vi "DG1022Z DVR.vi"(8 "error in (no error)":errorcluster, 10 "write buffer":string, 11 "VISA resource name":refnum<visa-resource-name>) -> (0 "error out":errorcluster, 2 "read buffer":string)   [LabVIEW 2025, in "Interface Functions.lvlib"]
uses:
  Interface Functions.lvlib
  <vilib>/Instr/_visa.llb/VISA Open Access Mode.ctl
  80e2d14e-0af9-4134-9fdb-927d146bfa2f.vi
  <vilib>/Utility/error.llb/Trim Whitespace One-Sided.vi
panel:
  out "Retries":i32
  out "read return count":u32
  out "write return count":u32
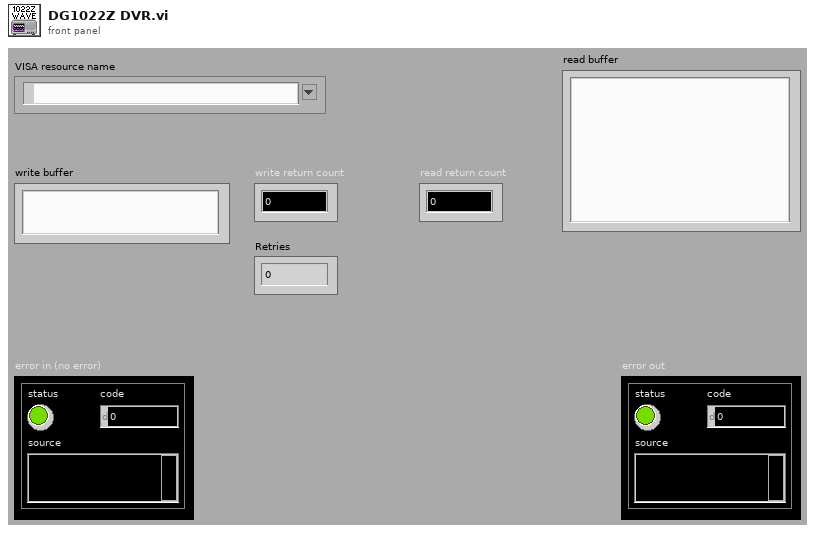
[diagram p1: front panel]
types:
  T1 = typedef "VISA Open Access Mode.ctl" = u32
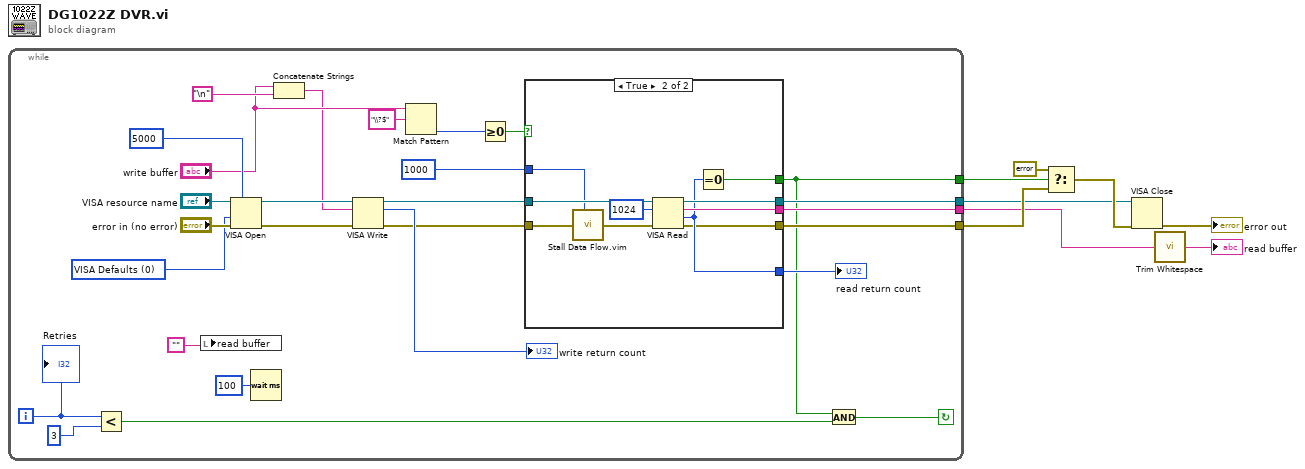
[diagram p0: block diagram]
diagram:
  n1 = while {
    tunnel: [w22] -> w5
    tunnel: [w14] -> w4
    tunnel: [w21] -> w3
    tunnel: [w18] -> w1
    i -> [w16]
    stop <- w12 continue-if-true
    w33 = T1 0 items=["VISA Defaults"=0, "Exclusive Lock"=1, "Load Configured Settings"=4] ("Access Mode")
    n2 = Less?(x=w16, y=3) -> (x < y?=w13:bool)
    n3 = local write "read buffer"("") -> ()
    n4 = VISA Open(timeout (0)=u32 5000 ("VISA Open timeout (0)"), access mode=w33, error in (no error)="error in (no error)", VISA resource name="VISA resource name") -> (VISA resource name=w30:refnum<visa-resource-name>, error out=w29:errorcluster)  [unwired: 1 in]
    n5 = Wait (ms)(milliseconds to wait=u32 100) -> ()  [unwired: 1 out]
    n6 = Concatenate Strings("write buffer", "\n") -> (w9:string)
    n7 = VISA Write(VISA resource name=w30, write buffer=w9, error in (no error)=w29) -> (VISA resource name out=w23:refnum<visa-resource-name>, return count=→"write return count":u32, error out=w19:errorcluster)
    n8 = Match Pattern(string="write buffer", regular expression="\\?$") -> (offset past match=w26:i32)  [unwired: 1 in, 3 out]
    n9 = Greater Or Equal To 0?(x=w26) -> (x >= 0?=w25:bool)
    n10 = case shown="True" w25 {
      tunnel: w23 -> [w37 w47]
      tunnel: w19 -> [w36 w38]
      tunnel: [w37 w45] -> w21
      tunnel: [_ w44] -> w18
      tunnel: [_ w43] -> w17
      tunnel: [w36 w42] -> w22
      tunnel: [_ w41] -> w14
      tunnel: u32 1000 ("milliseconds to wait") -> [_ w40]
      frame False {
      }
      frame True {
        n11 = call "Stall Data Flow.vim"("value in"=w38, "milliseconds to wait"=w40) -> ("value out"=w39:errorcluster)  [unwired: 1 out]
        n12 = VISA Read(VISA resource name=w47, byte count=u32 1024, error in (no error)=w39) -> (VISA resource name out=w45:refnum<visa-resource-name>, read buffer=w44:string, return count=w43:u32, error out=w42:errorcluster)
        n13 = Equal To 0?(x=w43) -> (x = 0?=w41:bool)
      }
    }
    "read return count" <- w17
    n14 = And(x=w14, y=w13) -> (x .and. y?=w12:bool)
    "Retries" <- w16
  }
  n15 = Select(t=errorcluster {"status"=FALSE, "code"=0, "source"=""}, s=w4, f=w5) -> (s? t:f=w6:errorcluster)
  n16 = VISA Close(VISA resource name=w3, error in (no error)=w6) -> (error out=→"error out":errorcluster)
  n17 = call <vilib>:"Trim Whitespace.vi"("string"=w1) -> ("trimmed string"=→"read buffer":string)  [unwired: 1 in]
